vi "Write Item Name.vi"(8 "error in (no error)":errorcluster, 10 "Item Name":string, 11 "Status in":refnum<class "Status.lvclass">) -> (0 "error out":errorcluster, 3 "Status out":refnum<class "Status.lvclass">)   [LabVIEW 2017, in "Message Interface.lvlib" / "Status.lvclass"]
uses:
  Status.lvclass
  Status.lvclass/Status.ctl
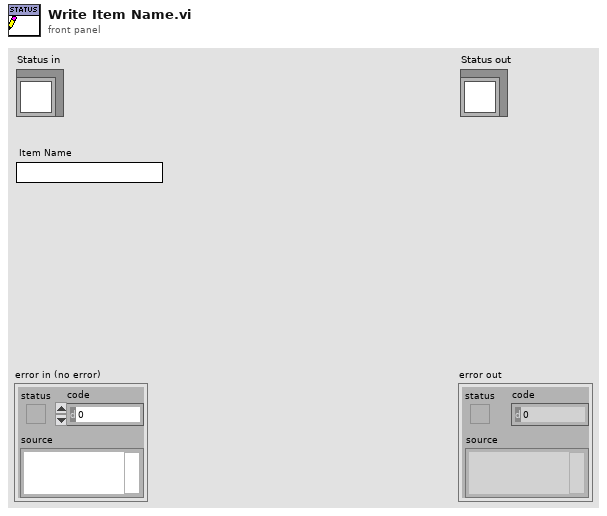
[diagram p1: front panel]
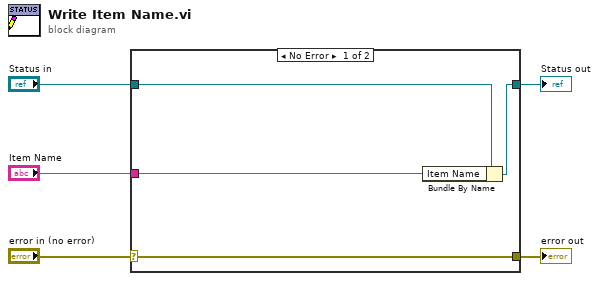
[diagram p0: block diagram]
diagram:
  n1 = case shown="No Error" "error in (no error)" {
    selector: "error in (no error)" -> [w9 w10]
    tunnel: [w9 w10] -> w4
    tunnel: [w7 w11] -> w2
    tunnel: "Status in" -> [w8 w11]
    tunnel: "Item Name" -> [w6 _]
    frame No Error {
      n2 = Bundle By Name(cluster=w8, "Item Name"=w6) -> (w7:refnum<class "Status.lvclass">)
    }
    frame Error {
    }
  }
  "error out" <- w4
  "Status out" <- w2
